vi "Intake Logic.vi"(1 "Operator Intake In":T3) -> (0 "Operator Intake Out":T3)   [LabVIEW 2013]
uses:
  <vilib>/Rock Robotics/WPI/Relay/WPI_RelayValue.ctl
  <vilib>/Rock Robotics/WPI/Solenoid/WPI_SolenoidValue.ctl
  Cannon/Cannon Global.vi
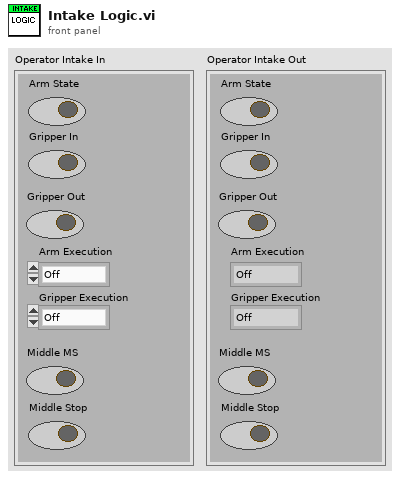
[diagram p1: front panel]
types:
  T1 = typedef "WPI_RelayValue.ctl" = enum16{"Off", "On", "Forward", "Reverse"}
  T2 = typedef "WPI_SolenoidValue.ctl" = enum16{"Off", "On", "Forward", "Reverse"}
  T3 = cluster{"Arm State":bool, "Gripper In":bool, "Gripper Out":bool, "Gripper Execution":T1, "Arm Execution":T2, "Middle MS":bool, "Middle Stop":bool}
  T4 = cluster{"Angle":dbl, "Clutch MS":bool, "Ball MS":bool, "Motor VBus":dbl, "Clutch ":T1, "LeFireatwill":bool, "Arm":bool, "Armed":bool, "Fire!":bool}
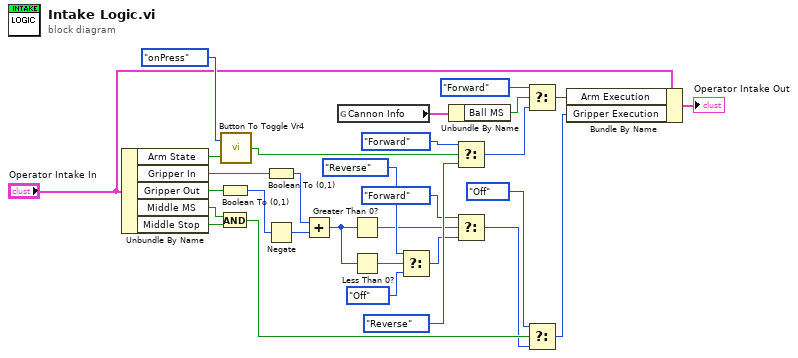
[diagram p0: block diagram]
diagram:
  n1 = Unbundle By Name("Operator Intake In") -> ("Arm State"=w29:bool, "Gripper In"=w25:bool, "Gripper Out"=w24:bool, "Middle MS"=w12:bool, "Middle Stop"=w11:bool)
  n2 = Boolean To (0,1)(Boolean=w24) -> (0, 1=w22:i16)
  n3 = And(x=w12, y=w11) -> (x .and. y?=w10:bool)
  n4 = call "Button To Toggle Vr4.vi"("InValue"=w29, "Action"=enum16{"onPress", "onRelease", "Both"}."onPress") -> ("Result"=w28:bool)
  n5 = Boolean To (0,1)(Boolean=w25) -> (0, 1=w23:i16)
  n6 = Negate(x=w22) -> (-x=w21:i16)
  n7 = Add(x=w23, y=w21) -> (x+y=w17:i16)
  n8 = global read "Cannon Global.vi" "Cannon Info"() -> (w2:T4)
  n9 = Greater Than 0?(x=w17) -> (x > 0?=w16:bool)
  n10 = Less Than 0?(x=w17) -> (x < 0?=w20:bool)
  n11 = Select(t=WPI_RelayValue."Reverse" ("Gripper Execution"), s=w20, f=WPI_RelayValue."Off" ("Gripper Execution")) -> (s? t:f=w15:T1)
  n12 = Unbundle By Name(w2) -> ("Ball MS"=w1:bool)
  n13 = Select(t=WPI_RelayValue."Forward" ("Gripper Execution"), s=w28, f=WPI_RelayValue."Reverse" ("Gripper Execution")) -> (s? t:f=w3:T1)
  n14 = Select(t=WPI_RelayValue."Forward" ("Gripper Execution"), s=w16, f=w15) -> (s? t:f=w9:T1)
  n15 = Select(t=WPI_RelayValue."Forward" ("Gripper Execution"), s=w1, f=w3) -> (s? t:f=w4:T1)
  n16 = Select(t=WPI_RelayValue."Off" ("Gripper Execution"), s=w10, f=w9) -> (s? t:f=w7:T1)
  n17 = Bundle By Name(cluster="Operator Intake In", "Arm Execution"=w4, "Gripper Execution"=w7) -> (→"Operator Intake Out":T3)
